vi "lux.vi"() -> ()   [LabVIEW 2020]
panel:
  out "lux":dbl
  in  "stop":bool
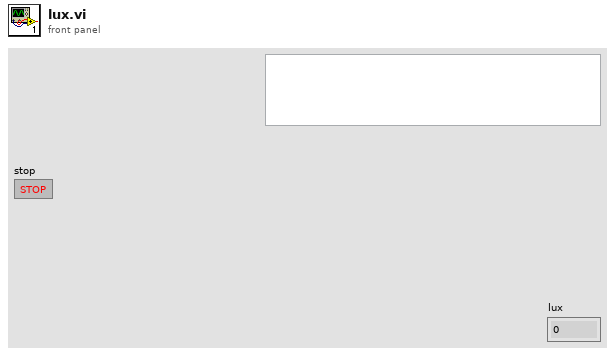
[diagram p1: front panel]
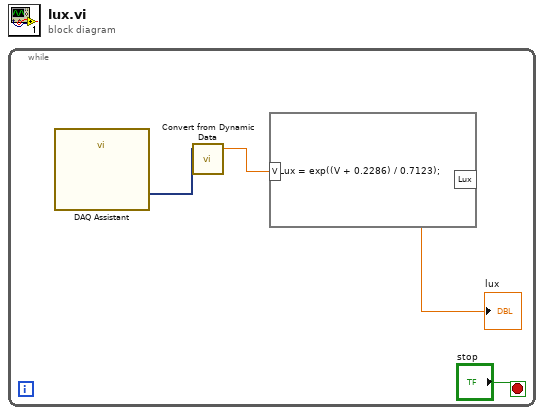
[diagram p0: block diagram]
diagram:
  n1 = while {
    stop <- "stop" stop-if-true
    n2 = call "DAQ Assistant"() -> ("data"=w1:dynamicdata)  [unwired: 17 in, 2 out]
    n3 = call "Convert from Dynamic Data"("Dynamic Data Type"=w1) -> ("Scalar"=w2:dbl)  [unwired: 3 in]
    n4 = formula code="Lux = exp((V + 0.2286) / 0.7123);"("V"=w2) -> ("Lux"=→"lux":dbl)
  }
